vi "PCO_GetCameraSynchMode.vi"(8 "error in (no error)":errorcluster {"code" format="%x"}, 11 "ph":u64) -> (0 "error out":errorcluster {"code" format="%x"}, 1 "wCameraSynchMode":u16(ring) items=["OFF", "MASTER", "SLAVE"], 2 "ErrorMessage":i32 format="%x", 3 "ph out":u64)   [LabVIEW 2019, in "SDK.lvlib" / "TimingControl.lvlib"]
doc: "<b>Description:</b>\nThis function returns the current camera synchronization mode. This Master / Slave synchronization mode is especially for multi-camera use.\nWhen cameras are cascaded through an external synchronization line at least one camera must be in master mode. This camera determines the timing of all other cameras in the line and therefore is the only camera, which accepts timing (exposure, delay,…) settings. All cameras which are set to slave mode synchronize its exposures with the master camera.\n\nTo get reliable results the follow start / stop rules should be observed:\nIn order to get the same number of images in the recorder, please set all slaves to Recording State [run] ((see PCO_GetRecordingState), before the master is set. When setting Recording State [stop] (see PCO_GetRecordingState), please stop the master as first. Please observe the start / stop sequence.\n\n<b>Supported camera type:</b>\npco.dimax\n\n<b>Descriptor dependency:</b>\ndwGeneralCaps3: CAMERA_SYNC"
uses:
  TimingControl.lvlib
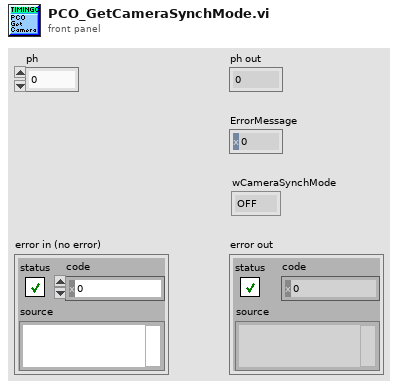
[diagram p1: front panel]
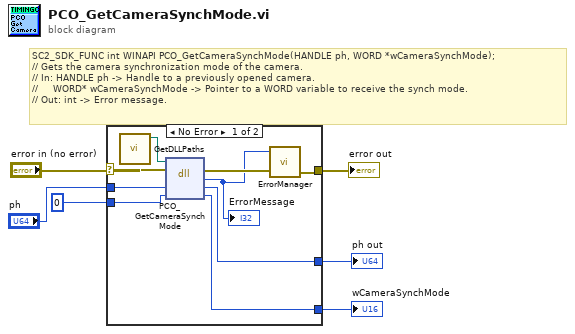
[diagram p0: block diagram]
diagram:
  # "SC2_SDK_FUNC int WINAPI PCO_GetCameraSynchMode(HANDLE ph, WORD *wCameraSynchMode);\n// Gets the camera synchronization mode of the camera.\n// In: HANDLE ph -> Handle to a previously opened camera.\n//     WORD* wCameraSynchMode -> Pointer to a WORD variable to receive the synch mode.\n// Out: int -> Error message."
  n1 = case shown="No Error" "error in (no error)" {
    selector: "error in (no error)" -> [w11 w18]
    tunnel: "ph" -> [w15 w17]
    tunnel: [w14 w17] -> w5
    tunnel: u16 0 ("wCameraSynchMode") -> [w13 w16]
    tunnel: [w12 w16] -> w3
    tunnel: [w9 w18] -> w2
    frame No Error {
      n2 = call "GetDLLPaths.vi"() -> ("SC2_Cam_Path"=w7:path)  [unwired: 9 in, 2 out]
      n3 = dll-call lib="?" fn="PCO_GetCameraSynchMode"(path in=w7, error in=w11, "ph"=w15, "wCameraSynchMode"=w13) -> (error out=w10:errorcluster, "return type"=w8:i32, "ph"=w14:u64, "wCameraSynchMode"=w12:u16)  [unwired: 1 in, 1 out]
      "ErrorMessage" <- w8
      n4 = call "ErrorManager.vi"("error in (no error)"=w10, "error code"=w8) -> ("error out"=w9:errorcluster)  [unwired: 3 in]
    }
    frame Error {
    }
  }
  "ph out" <- w5
  "wCameraSynchMode" <- w3
  "error out" <- w2
